vi "Restaurante.vi"() -> ()   [LabVIEW 2015]
panel:
  out "Numeric":dbl
  out "LedMesas":T1
  out "DESCRIPCION COMANDA":string[][](array[string])
  in  "Salir":bool
  in  "MENU":T2
  in  "MESAS":T3
  in  "CerrarComanda":bool
  in  "Modif.Comanda":bool
  in  "NuevaComanda":bool
  # "Descripcion"
  # "Precio"
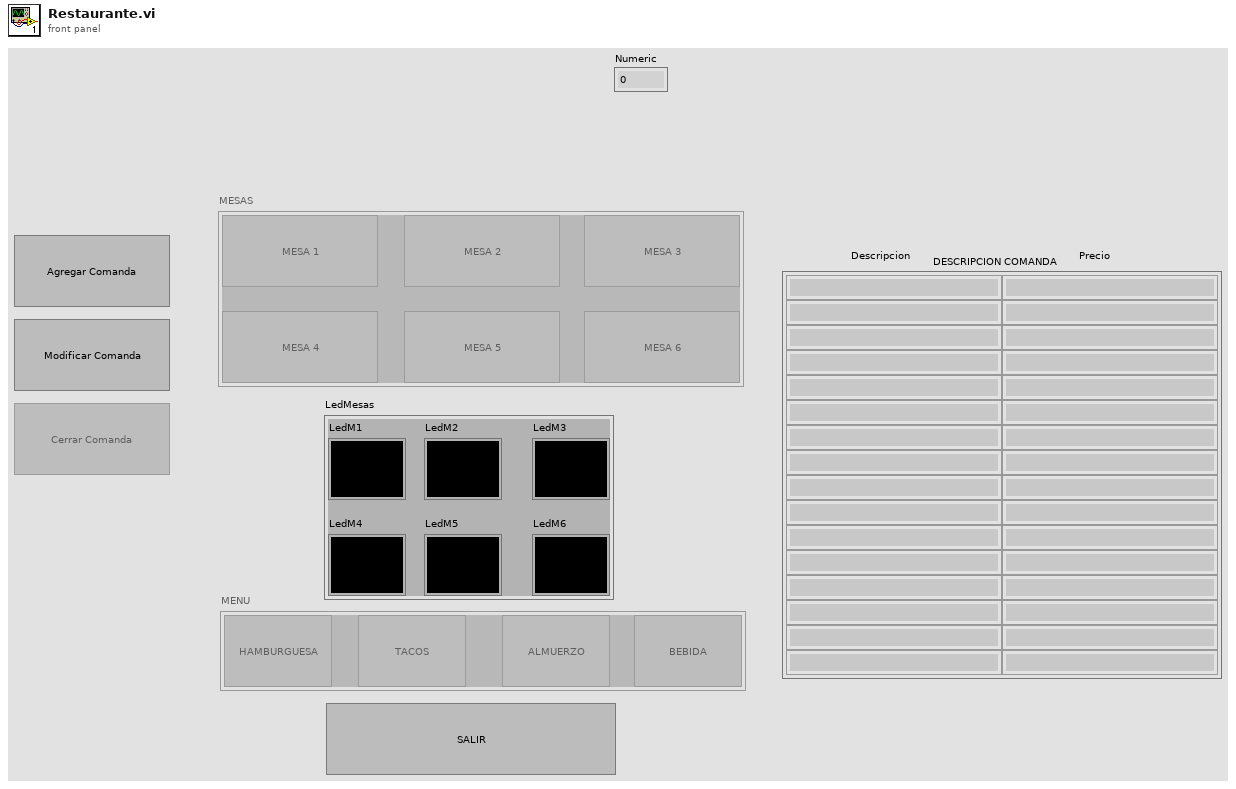
[diagram p1: front panel]
types:
  T1 = cluster{"LedM1":bool, "LedM2":bool, "LedM3":bool, "LedM4":bool, "LedM5":bool, "LedM6":bool}
  T2 = cluster{"Ham":bool, "Tacos":bool, "Almuerzo":bool, "Bebida":bool}
  T3 = cluster{"M1":bool, "M2":bool, "M3":bool, "M4":bool, "M5":bool, "M6":bool}
  T4 = enum8{"Enabled", "Disabled", "Disabled and Grayed Out"}
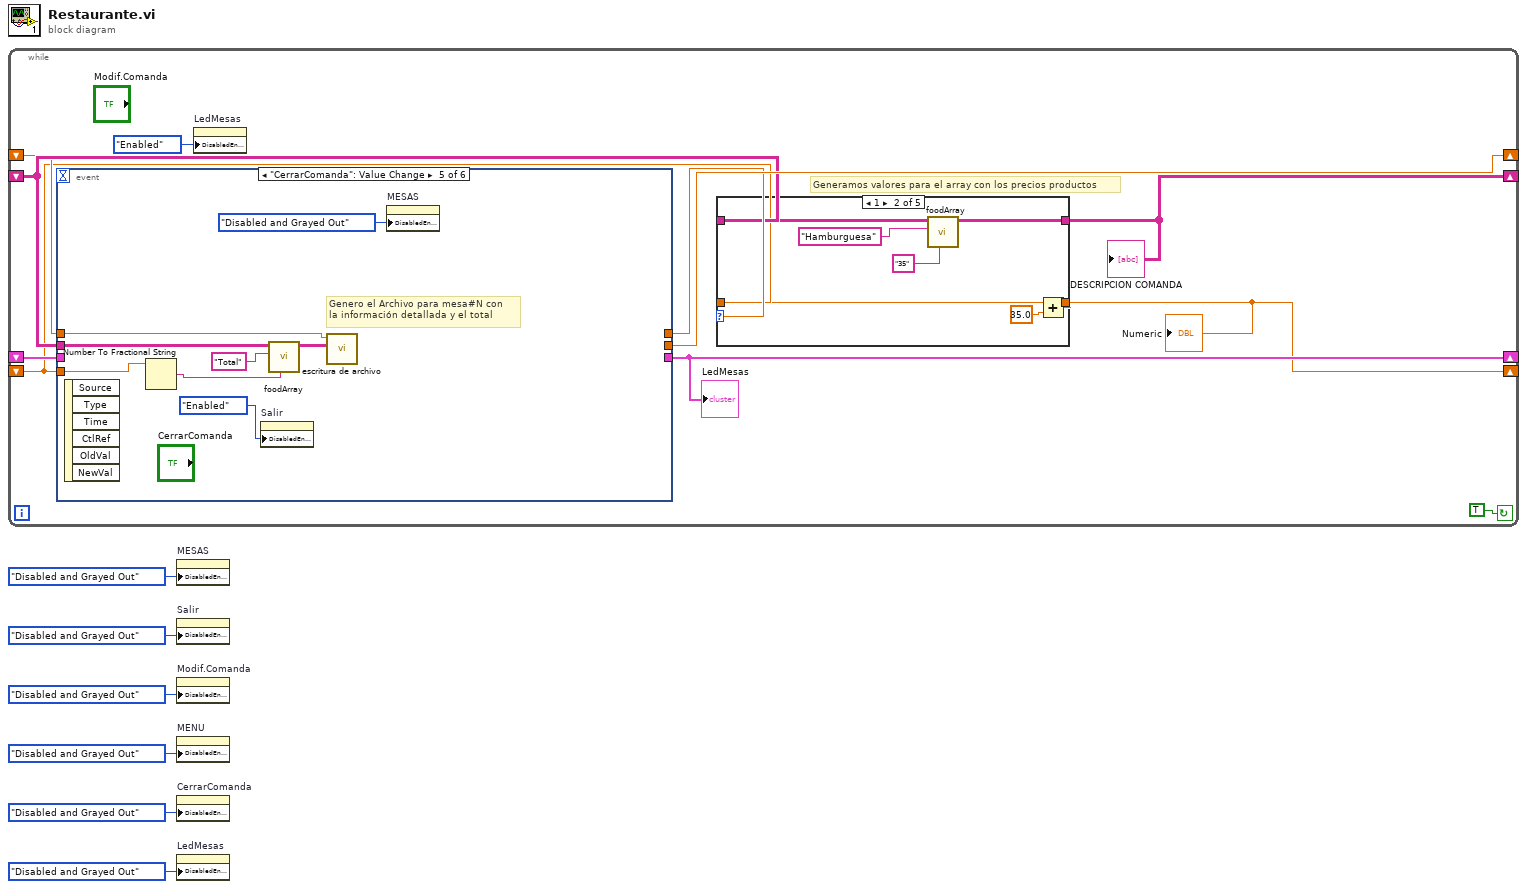
[diagram p0: block diagram]
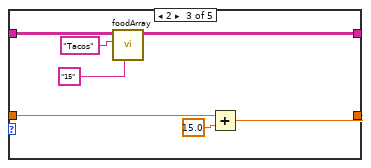
[diagram p3: hidden frame]
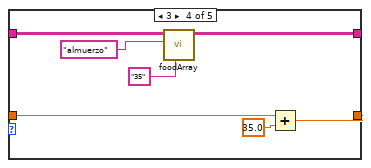
[diagram p4: hidden frame]
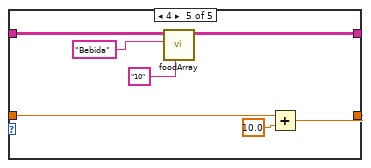
[diagram p5: hidden frame]
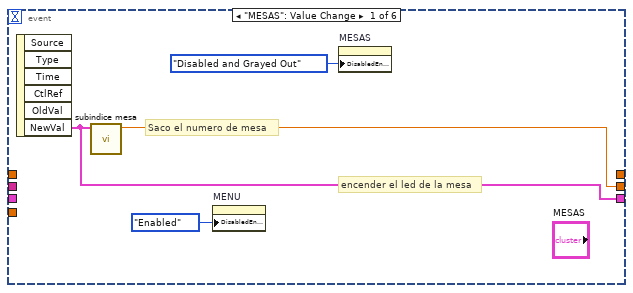
[diagram p6: hidden frame]
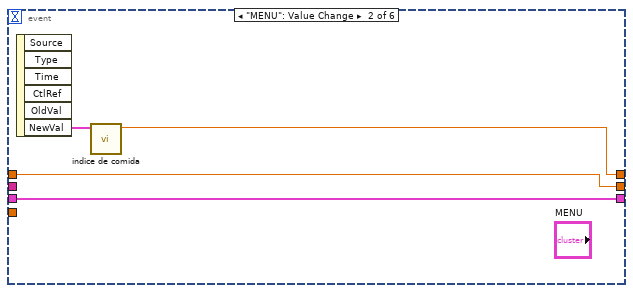
[diagram p7: hidden frame]
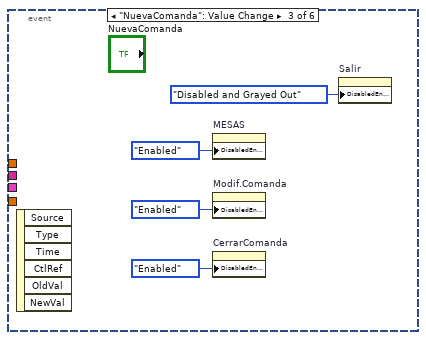
[diagram p8: hidden frame]
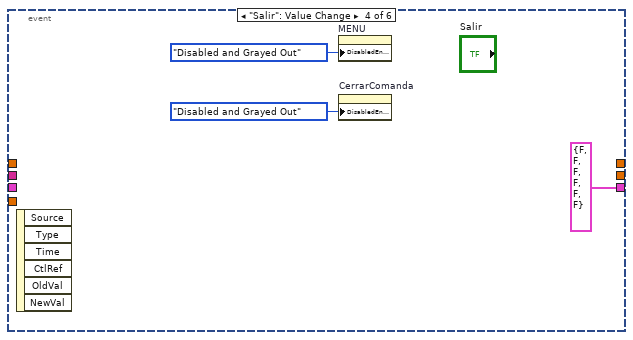
[diagram p9: hidden frame]
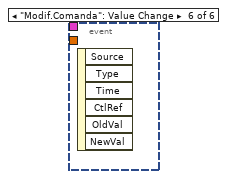
[diagram p10: hidden frame]
diagram:
  n1 = while {
    shift-right: [w17] -> _
    shift-left: _ -> [w9]
    shift-right: [w14] -> _
    shift-left: _ -> [w12]
    shift-right: [w11] -> _
    shift-left: _ -> [w10]
    shift-right: [w8] -> _
    shift-left: _ -> [w7]
    stop <- TRUE continue-if-true
    # "Generamos valores para el array con los precios productos"
    n2 = event shown="[4] \"CerrarComanda\": Value Change" {
      selector: _ -> [_ _ _ _ _ _]
      dyn-events: _ -> [_ _ _ _ _ _]
      timeout: _ -> [_ _ _ _ _ _]
      tunnel: [w49 w52 _ _ _ _] -> w17
      tunnel: [_ w54 _ _ _ _] -> w15
      tunnel: [w48 w53 _ T1 {"LedM1"=FALSE, "LedM2"=FALSE, "LedM3"=FALSE, "LedM4"=FALSE, "LedM5"=FALSE, "LedM6"=FALSE} ("LedMesas") _ _] -> w11
      tunnel: w12 -> [_ _ _ _ w67 _]
      tunnel: w10 -> [_ w53 _ _ _ _]
      tunnel: w9 -> [_ w52 _ _ w68 _]
      tunnel: w7 -> [_ _ _ _ w65 _]
      event "MESAS": Value Change {
        # "encender el led de la mesa"
        # "Saco el numero de mesa"
        n3 = event-data() -> ("NewVal"=w48:T3)  [unwired: 1 in, 5 out]
        n4 = call "subindice mesa.vi"("NewVal"=w48) -> ("Numeric"=w49:dbl)  [unwired: 10 in]
        n5 = property on="MENU" class="Clust"("DisabledEnum"=T4."Enabled" ("Disabled")) -> ()  [unwired: 2 in, 2 out]
        n6 = property on="MESAS" class="Clust"("DisabledEnum"=T4."Disabled and Grayed Out" ("Disabled")) -> ()  [unwired: 2 in, 2 out]
      }
      event "MENU": Value Change {
        n7 = event-data() -> ("NewVal"=w55:T2)  [unwired: 1 in, 5 out]
        n8 = call "indice de comida.vi"("NewVal"=w55) -> ("Numeric"=w54:dbl)  [unwired: 10 in]
      }
      event "NuevaComanda": Value Change {
        n9 = event-data() -> ()  [unwired: 1 in, 6 out]
        n10 = property on="MESAS" class="Clust"("DisabledEnum"=T4."Enabled" ("Disabled")) -> ()  [unwired: 2 in, 2 out]
        n11 = property on="Modif.Comanda" class="Bool"("DisabledEnum"=T4."Enabled" ("Disabled")) -> ()  [unwired: 2 in, 2 out]
        n12 = property on="CerrarComanda" class="Bool"("DisabledEnum"=T4."Enabled" ("Disabled")) -> ()  [unwired: 2 in, 2 out]
        n13 = property on="Salir" class="Bool"("DisabledEnum"=T4."Disabled and Grayed Out" ("Disabled")) -> ()  [unwired: 2 in, 2 out]
      }
      event "Salir": Value Change {
        n14 = event-data() -> ()  [unwired: 1 in, 6 out]
        n15 = property on="MENU" class="Clust"("DisabledEnum"=T4."Disabled and Grayed Out" ("Disabled")) -> ()  [unwired: 2 in, 2 out]
        n16 = property on="CerrarComanda" class="Bool"("DisabledEnum"=T4."Disabled and Grayed Out" ("Disabled")) -> ()  [unwired: 2 in, 2 out]
      }
      event "CerrarComanda": Value Change {
        # "Genero el Archivo para mesa#N con\nla información detallada y el total"
        n17 = event-data() -> ()  [unwired: 1 in, 6 out]
        n18 = Number To Fractional String(number=w65) -> (F-format string=w64:string)  [unwired: 3 in]
        n19 = property on="Salir" class="Bool"("DisabledEnum"=T4."Enabled" ("Disabled")) -> ()  [unwired: 2 in, 2 out]
        n20 = call "foodArray.vi"("element"=w64, "element 2"="Total", "Array in"=w67) -> ("Array out"=w63:string[][])  [unwired: 8 in]
        n21 = call "escritura de archivo.vi"("Array in"=w63, "Numeric"=w68) -> ()  [unwired: 10 in]
        n22 = property on="MESAS" class="Clust"("DisabledEnum"=T4."Disabled and Grayed Out" ("Disabled")) -> ()  [unwired: 2 in, 2 out]
      }
      event "Modif.Comanda": Value Change {
        n23 = event-data() -> ()  [unwired: 1 in, 6 out]
      }
    }
    "LedMesas" <- w11
    n24 = property on="LedMesas" class="Clust (strict)"("DisabledEnum"=T4."Enabled" ("Disabled")) -> ()  [unwired: 2 in, 2 out]
    n25 = case shown="1" w15 {
      tunnel: [w19 w26 w30 w39 w45] -> w14
      tunnel: w12 -> [w19 w23 w33 w40 w47]
      tunnel: [w18 w22 w27 w34 w41] -> w8
      tunnel: w7 -> [w18 w21 w28 w35 w42]
      frame 0, Default {
      }
      frame 1 {
        n26 = call "foodArray.vi"("element"="35", "element 2"="Hamburguesa", "Array in"=w23) -> ("Array out"=w26:string[][])  [unwired: 8 in]
        n27 = Add(x=w21, y=35.0) -> (x+y=w22:dbl)
      }
      frame 2 {
        n28 = call "foodArray.vi"("element"="15", "element 2"="Tacos", "Array in"=w33) -> ("Array out"=w30:string[][])  [unwired: 8 in]
        n29 = Add(x=w28, y=15.0) -> (x+y=w27:dbl)
      }
      frame 3 {
        n30 = call "foodArray.vi"("element"="35", "element 2"="almuerzo", "Array in"=w40) -> ("Array out"=w39:string[][])  [unwired: 8 in]
        n31 = Add(x=w35, y=35.0) -> (x+y=w34:dbl)
      }
      frame 4 {
        n32 = call "foodArray.vi"("element"="10", "element 2"="Bebida" ("element"), "Array in"=w47) -> ("Array out"=w45:string[][])  [unwired: 8 in]
        n33 = Add(x=w42, y=10.0) -> (x+y=w41:dbl)
      }
    }
    "DESCRIPCION COMANDA" <- w14
    "Numeric" <- w8
  }
  n34 = property on="MESAS" class="Clust"("DisabledEnum"=T4."Disabled and Grayed Out" ("Disabled")) -> ()  [unwired: 2 in, 2 out]
  n35 = property on="Salir" class="Bool"("DisabledEnum"=T4."Disabled and Grayed Out" ("Disabled")) -> ()  [unwired: 2 in, 2 out]
  n36 = property on="Modif.Comanda" class="Bool"("DisabledEnum"=T4."Disabled and Grayed Out" ("Disabled")) -> ()  [unwired: 2 in, 2 out]
  n37 = property on="MENU" class="Clust"("DisabledEnum"=T4."Disabled and Grayed Out" ("Disabled")) -> ()  [unwired: 2 in, 2 out]
  n38 = property on="CerrarComanda" class="Bool"("DisabledEnum"=T4."Disabled and Grayed Out" ("Disabled")) -> ()  [unwired: 2 in, 2 out]
  n39 = property on="LedMesas" class="Clust (strict)"("DisabledEnum"=T4."Disabled and Grayed Out" ("Disabled")) -> ()  [unwired: 2 in, 2 out]
